vi "tearDown.vi"(8 "error in (no error)":errorcluster, 11 "reference in":refnum<class "TestTextFileSink.lvclass">) -> (0 "error out":errorcluster, 3 "reference out":refnum<class "TestTextFileSink.lvclass">)   [LabVIEW 2017, in "TestTextFileSink.lvclass"]
doc: "tearDown runs after the test method has completed. Use this method to clean up any operations or references that were opened by setUp or the test method. Unit tests should be independent of other unit tests so this VI should ensure that the next test can run in a 'clean' test environment."
uses:
  TestTextFileSink.lvclass
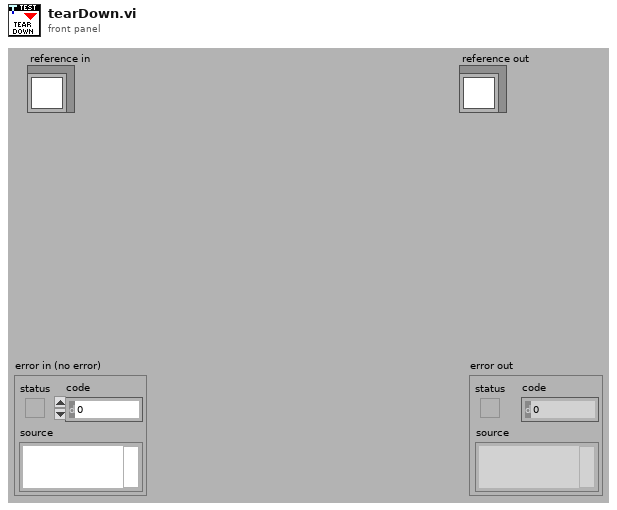
[diagram p1: front panel]
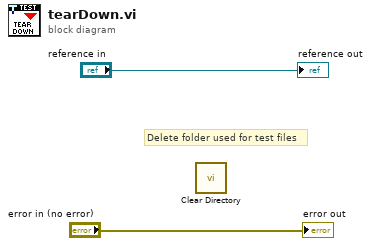
[diagram p0: block diagram]
diagram:
  # "Delete folder used for test files"
  n1 = call "Clear Directory.vi"() -> ()  [unwired: 11 in, 1 out]
  "error out" <- "error in (no error)"
  "reference out" <- "reference in"
